vi "rwfm_CreateChan.vi"(8 "error in":errorcluster, 10 "Sensitivity":sgl[](array[numeric]), 11 "Dynamic FPGA VI Reference":T1) -> (0 "error out":errorcluster, 3 "Dynamic FPGA VI Reference":T1)   [LabVIEW 2017, in "cRIOWfmLibMcsa.lvlib"]
doc: "This VI collects and sends scaling coefficients as well as channel count to the FPGA. The number of elements in \"Channel Info\" must equal the number of channels acquired by the FPGA."
uses:
  <vilib>/addons/InsightCM/Devices/Shared/Mcsa/cRIOWfmAcqMcsa/cRIOWfmLibMcsa.lvlib
  <vilib>/addons/InsightCM/Devices/Shared/Mcsa/cRIOWfmAcqMcsa/controls/rwfm_DynamicFPGArefMCSA.ctl
  <vilib>/Utility/error.llb/Error Cluster From Error Code.vi
  <vilib>/rvi/errors/niLvFpgaAdjustHostInterfaceError.vi
  <vilib>/rvi/interface/nirviReadWriteControl/nirviReadWriteControl.xnode
  <vilib>/rvi/interface/Simulation/niFpgaSimulationCallBeginRW.vi
  NiFpgaLv.dll
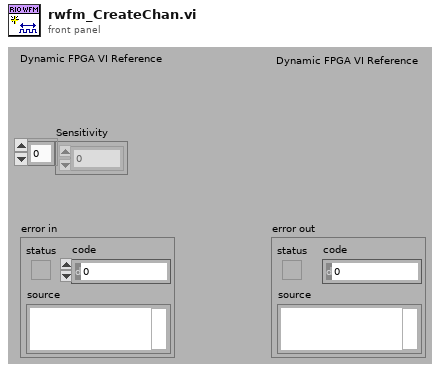
[diagram p1: front panel]
types:
  T1 = typedef "cRIOWfmLibMcsa.lvlib/rwfm_DynamicFPGArefMCSA.ctl" = refnum<k20>
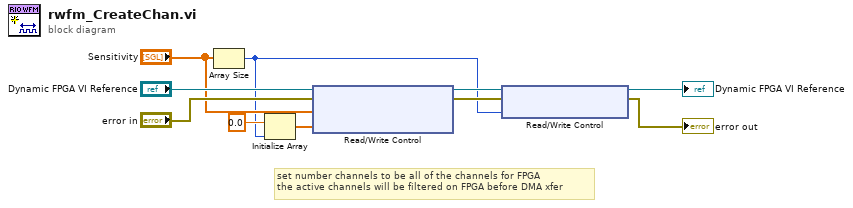
[diagram p0: block diagram]
diagram:
  # "set number channels to be all of the channels for FPGA\nthe active channels will be filtered on FPGA before DMA xfer"
  n1 = Array Size(array="Sensitivity") -> (size(s)=w1:i32)
  n2 = Initialize Array(sgl 0.0, w1) -> (w4:sgl[])
  n3 = xnode "Read/Write Control"("FPGA VI Reference In"="Dynamic FPGA VI Reference", "error in"="error in", "Custom Scale Slope"="Sensitivity", "Custom Scale Intercept"=w4) -> ("FPGA VI Reference Out"=w9:T1, "error out"=w8:errorcluster)
  n4 = xnode "Read/Write Control"("FPGA VI Reference In"=w9, "error in"=w8, "Total Avail Channels"=w1) -> ("FPGA VI Reference Out"=→"Dynamic FPGA VI Reference":T1, "error out"=→"error out":errorcluster)
